vi "Destroy.vi"(8 "ErrorIn":errorcluster, 11 "ReferenceIn":refnum<class "DemoApplication.lvclass">) -> (0 "ErrorOut":errorcluster, 3 "ReferenceOut":refnum<class "DemoApplication.lvclass">)   [LabVIEW 2021, in "DemoApplication.lvclass"]
doc: "Destroy the object instance"
uses:
  DemoApplication.lvclass
  .Externals/Library_TAF_ApplicationFramework/MasterGUI/MasterGUI.lvclass
  DemoApplication.lvclass/DemoApplication.ctl
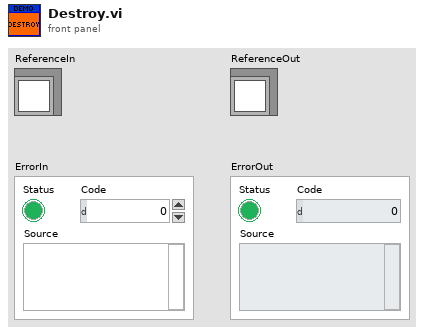
[diagram p1: front panel]
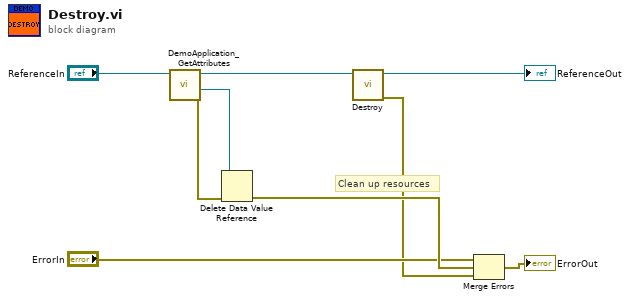
[diagram p0: block diagram]
diagram:
  # "Clean up resources"
  n1 = call "DemoApplication_GetAttributes.vi"("ReferenceIn"="ReferenceIn") -> ("ErrorOut"=w8:errorcluster, "DataRef"=w3:refnum<data-value>, "ReferenceOut"=w4:refnum<class "DemoApplication.lvclass">)  [unwired: 7 in, 1 out]
  n2 = Delete Data Value Reference(data value reference=w3, error in=w8) -> (error out=w7:errorcluster)  [unwired: 1 out]
  n3 = call-parent "Destroy.vi"("ReferenceIn"=w4) -> ("ErrorOut"=w5:errorcluster, "ReferenceOut"=→"ReferenceOut":refnum<class "DemoApplication.lvclass">)  [unwired: 9 in]
  n4 = Merge Errors("ErrorIn", w7, w5) -> (→"ErrorOut":errorcluster)
